vi "AdaptToInputs.vi"(3 "Term Types":T1, 4 "XRef":refnum<vi>, 5 "State In":T5) -> (0 "Reply":string[](array[string]), 2 "State Out":T5)   [LabVIEW 2018, in "Shuffle Array.xnode"]
uses:
  Shuffle Array.xnode
  State.ctl
  <vilib>/XNodeSupport/XNodeTermTypeIDPairs.ctl
  <vilib>/XNodeSupport/XNodeTermTypeIDPair.ctl
  <vilib>/XNodeSupport/XNodeType.ctl
  <vilib>/XNodeSupport/XNodeString.ctl
  <userlib>/_LAVAcr/Scripting Tools/XNode Support/TypeDefs/Array Dimension Tests.ctl
  <userlib>/_LAVAcr/Scripting Tools/XNode Support/Find term type by ID_type.vi
  <userlib>/_LAVAcr/Scripting Tools/XNode Support/XNode Support.lvlib
  <vilib>/XNodeSupport/NI_XNodeSupport.lvlib
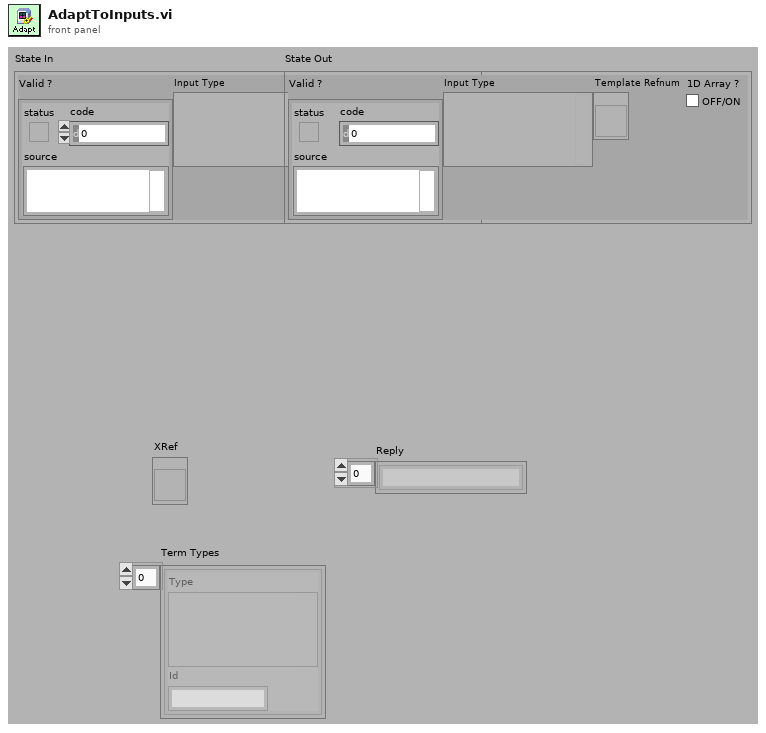
[diagram p1: front panel]
types:
  T1 = typedef "NI_XNodeSupport.lvlib/XNodeTermTypeIDPairs.ctl" = T2[]
  T2 = typedef "NI_XNodeSupport.lvlib/XNodeTermTypeIDPair.ctl" = cluster{"Type":T3, "Id":T4}
  T3 = typedef "NI_XNodeSupport.lvlib/XNodeType.ctl" = variant
  T4 = typedef "NI_XNodeSupport.lvlib/XNodeString.ctl" = string
  T5 = typedef "Shuffle Array.xnode/State.ctl" = cluster{"Valid ?":errorcluster, "Input Type":variant, "Template Refnum":refnum<vi>, "1D Array ?":bool}
  T6 = typedef "Scripting Tools.lvlib/XNode Support.lvlib/Array Dimension Tests.ctl" = enum16{"No Check", "At Least n dimensions", "Exactly N Dimensions", "No More Than N Dimensions"}
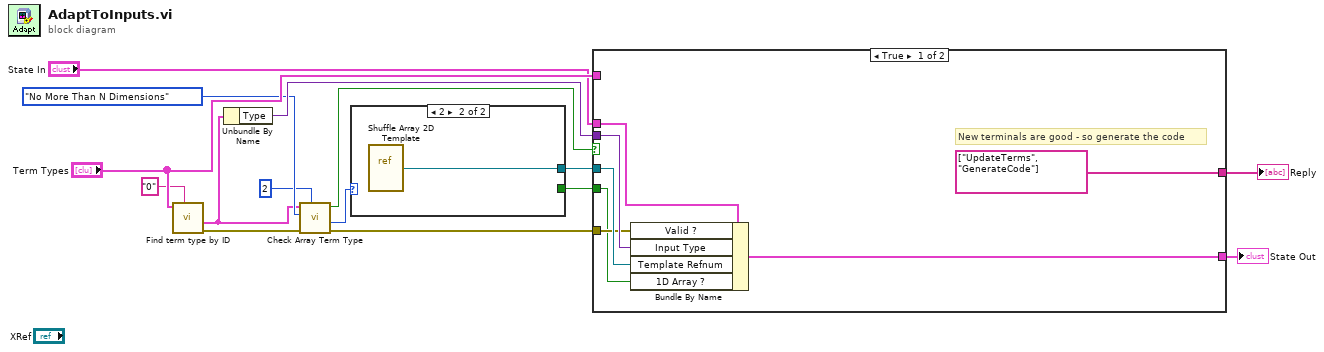
[diagram p0: block diagram]
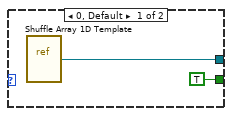
[diagram p2: hidden frame]
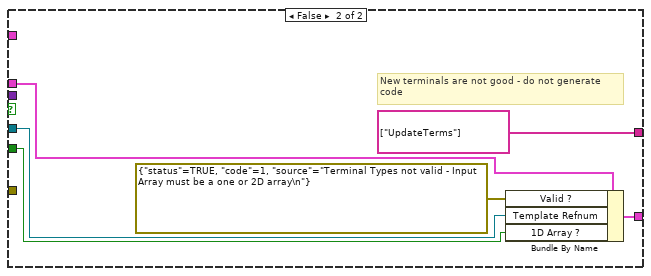
[diagram p3: hidden frame]
diagram:
  n1 = call-poly <userlib>:"Find term type by ID.vi"("Search ID"="0", "Term Types"="Term Types") -> ("error out"=w5:errorcluster, "Term Type"=w1:T2)  [unwired: 1 in, 7 out]
  n2 = Unbundle By Name(w1) -> ("Type"=w10:T3)
  n3 = call <userlib>:"Check Array Term Type.vi"("Dimensions Required"=2, "error in (no error)"=w5, "Dimension Check"=Array_Dimension_Tests."No More Than N Dimensions", "Term Type"=w1) -> ("error out"=w8:errorcluster, "Array Dimensions"=w2:i32, "Is Good ?"=w15:bool)  [unwired: 1 in, 4 out]
  n4 = case shown="2" w2 {
    tunnel: [w17 w18] -> w9
    tunnel: [TRUE _] -> w7
    frame 0, Default {
      n5 = vi-ref "Shuffle Array 1D Template.vi"() -> (w17:refnum<vi>)
    }
    frame 2 {
      n6 = vi-ref "Shuffle Array 2D Template.vi"() -> (w18:refnum<vi>)
    }
  }
  n7 = case shown="True" w15 {
    tunnel: "Term Types" -> [_ _]
    tunnel: "State In" -> [w25 w31]
    tunnel: [w24 w29] -> w12
    tunnel: [string[] ["UpdateTerms", "GenerateCode"] ("Reply") string[] ["UpdateTerms"] ("Reply")] -> w11
    tunnel: w10 -> [w22 _]
    tunnel: w9 -> [w21 w27]
    tunnel: w8 -> [w20 _]
    tunnel: w7 -> [w19 w26]
    frame True {
      # "New terminals are good - so generate the code"
      n8 = Bundle By Name(cluster=w25, "Valid ?"=w20, "Input Type"=w22, "Template Refnum"=w21, "1D Array ?"=w19) -> (w24:T5)
    }
    frame False {
      # "New terminals are not good - do not generate\ncode"
      n9 = Bundle By Name(cluster=w31, "Valid ?"=errorcluster {"status"=TRUE, "code"=1, "source"="Terminal Types not valid - Input Array must be a one or 2D array\n"}, "Template Refnum"=w27, "1D Array ?"=w26) -> (w29:T5)
    }
  }
  "Reply" <- w11
  "State Out" <- w12
